vi "Read.vi"(8 "error in (no error)":errorcluster, 9 "Starting independent variables":dbl[](array[numeric]), 10 "Current independent variables":dbl[](array[numeric]), 11 "LCD Reader in":refnum<class "LCD Reader.lvclass">) -> (0 "error out":errorcluster, 2 "Data Channels":T1, 3 "LCD Reader out":refnum<class "LCD Reader.lvclass">)   [LabVIEW 2012, in "LCD Reader.lvclass"]
doc: "Prepare for read, wait the time delay, and take data from up to 4 channels."
uses:
  LCD Reader.lvclass
  Instruments/Utility Classes/Readable/Data Channels.ctl
  Instruments/Utility Classes/Readable/Data Channel.ctl
  Instruments/Utility Classes/Readable/Data Point.ctl
  Instruments/Utility Classes/Readable/Time.ctl
  Instruments/Utility Classes/Readable/X.ctl
  Instruments/LCD/LCD Retarder.lvclass
  LCD Reader.lvclass/LCD Reader.ctl
  Reader/Reader.lvclass
  Instruments/Utility Classes/Readable/Readable.lvclass
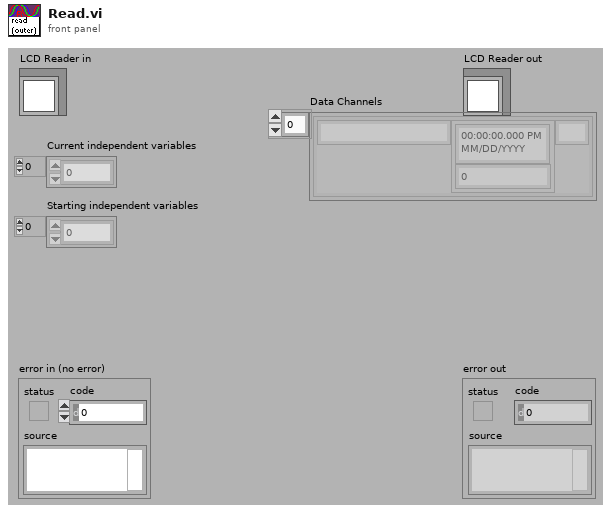
[diagram p1: front panel]
types:
  T1 = typedef "Readable.lvclass/Data Channels.ctl" = T2[]
  T2 = typedef "Readable.lvclass/Data Channel.ctl" = cluster{"Name":string, "Data Point":T3, "Unit":string}
  T3 = typedef "Readable.lvclass/Data Point.ctl" = cluster{"t":T4, "x":T5}
  T4 = typedef "Readable.lvclass/Time.ctl" = timestamp
  T5 = typedef "Readable.lvclass/X.ctl" = dbl
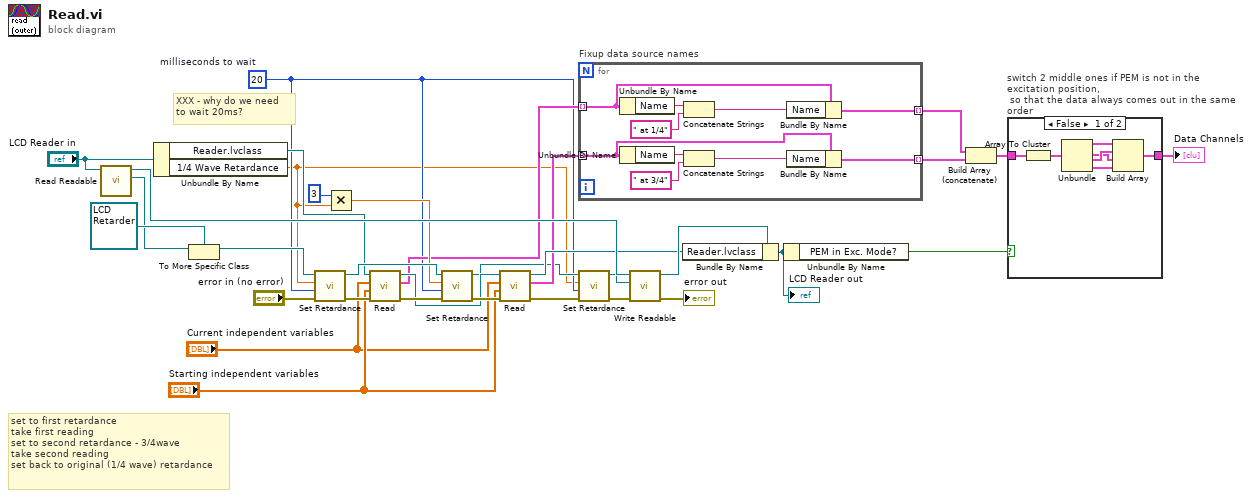
[diagram p0: block diagram]
diagram:
  w6 = u32 20  # milliseconds to wait
  # "XXX - why do we need\nto wait 20ms?"
  # "set to first retardance\ntake first reading\nset to second retardance - 3/4wave\ntake second reading\nset back to original (1/4 wave) retardance"
  n1 = call-dynamic "Read Readable.vi"("Reader.lvclass in"="LCD Reader in") -> ("Readable.lvclass"=w29:refnum<class "Readable.lvclass">, "Reader.lvclass out"=w25:refnum<class "LCD Reader.lvclass">)  [unwired: 1 in, 8 out]
  n2 = Unbundle By Name("LCD Reader in") -> ("Reader.lvclass"=w21:refnum<class "Reader.lvclass">, "1/4 Wave Retardance"=w3:dbl[unit])
  n3 = To More Specific Class(target class=refnum<class "LCD Retarder.lvclass"> refnum ("LCD Retarder.lvclass"), reference=w29) -> (specific class reference=w28:refnum<class "LCD Retarder.lvclass">)  [unwired: 1 in, 1 out]
  n4 = call "Set Retardance.vi"("errorIN"="error in (no error)", "milliseconds to wait (0)"=w6, "Retardance"=w3, "LCD in"=w28) -> ("errorOUT"=w27:errorcluster, "LCD out"=w31:refnum<class "LCD Retarder.lvclass">)  [unwired: 6 out]
  n5 = Multiply(x=3, y=w3) -> (x*y=w14:dbl[unit])
  n6 = call-dynamic "Read.vi"("error in (no error)"=w27, "Starting independent variables"="Starting independent variables", "Current independent variables"="Current independent variables", "Reader in"=w21) -> ("error out"=w26:errorcluster, "Data Channels"=w13:T1, "Reader out"=w23:refnum<class "Reader.lvclass">)  [unwired: 5 out]
  n7 = call "Set Retardance.vi"("errorIN"=w26, "milliseconds to wait (0)"=w6, "Retardance"=w14, "LCD in"=w31) -> ("errorOUT"=w24:errorcluster, "LCD out"=w9:refnum<class "LCD Retarder.lvclass">)  [unwired: 6 out]
  n8 = call-dynamic "Read.vi"("error in (no error)"=w24, "Starting independent variables"="Starting independent variables", "Current independent variables"="Current independent variables", "Reader in"=w23) -> ("error out"=w7:errorcluster, "Data Channels"=w12:T1, "Reader out"=w19:refnum<class "Reader.lvclass">)  [unwired: 5 out]
  n9 = for "Fixup data source names" {
    tunnel: w13 -> [w36] mode=indexing
    tunnel: w12 -> [w39] mode=indexing
    tunnel: [w38] -> w11 mode=indexing
    tunnel: [w34] -> w10 mode=indexing
    n10 = Unbundle By Name(w36) -> ("Name"=w40:string)
    n11 = Unbundle By Name(w39) -> ("Name"=w43:string)
    n12 = Concatenate Strings(w40, " at 1/4" ("string")) -> (w35:string)
    n13 = Concatenate Strings(w43, " at 3/4" ("string")) -> (w37:string)
    n14 = Bundle By Name(cluster=w36, "Name"=w35) -> (w34:T2)
    n15 = Bundle By Name(cluster=w39, "Name"=w37) -> (w38:T2)
  }
  n16 = call "Set Retardance.vi"("errorIN"=w7, "milliseconds to wait (0)"=w6, "Retardance"=w3, "LCD in"=w9) -> ("errorOUT"=w5:errorcluster, "LCD out"=w8:refnum<class "LCD Retarder.lvclass">)  [unwired: 6 out]
  n17 = call-dynamic "Write Readable.vi"("error in (no error)"=w5, "Readable.lvclass"=w8, "Reader.lvclass in"=w25) -> ("error out"=→"error out":errorcluster, "Reader.lvclass out"=w20:refnum<class "LCD Reader.lvclass">)  [unwired: 7 out]
  n18 = Bundle By Name(cluster=w20, "Reader.lvclass"=w19) -> (w16:refnum<class "LCD Reader.lvclass">)
  "LCD Reader out" <- w16
  n19 = Unbundle By Name(w16) -> ("PEM in Exc. Mode?"=w15:bool)
  n20 = Build Array (concatenate)(w10, w11) -> (w33:T2[])
  n21 = case "switch 2 middle ones if PEM is not in the excitation position,\n so that the data always comes out in the same order" shown="False" w15 {
    tunnel: w33 -> [w50 w51]
    tunnel: [w46 w51] -> w18
    frame False {
      n22 = Array To Cluster(array=w50) -> (cluster=w49:cluster{"[0]":T2, "[1]":T2, "[2]":T2, "[3]":T2})
      n23 = Unbundle(w49) -> ("[0]"=w48:T2, "[1]"=w44:T2, "[2]"=w45:T2, "[3]"=w47:T2)
      n24 = Build Array(w48, w45, w44, w47) -> (w46:T2[])
    }
    frame True {
    }
  }
  "Data Channels" <- w18
